vi "judge.vi"(5 "alpha":dbl, 6 "c_y":dbl, 7 "c_x":dbl, 8 "Original Plots":T1(array[cluster]), 9 "dy":dbl, 10 "dx":dbl, 11 "Captured Plots":T1(array[cluster])) -> (0 "result":bool)   [LabVIEW 2012]
panel:
  out "counter":i32
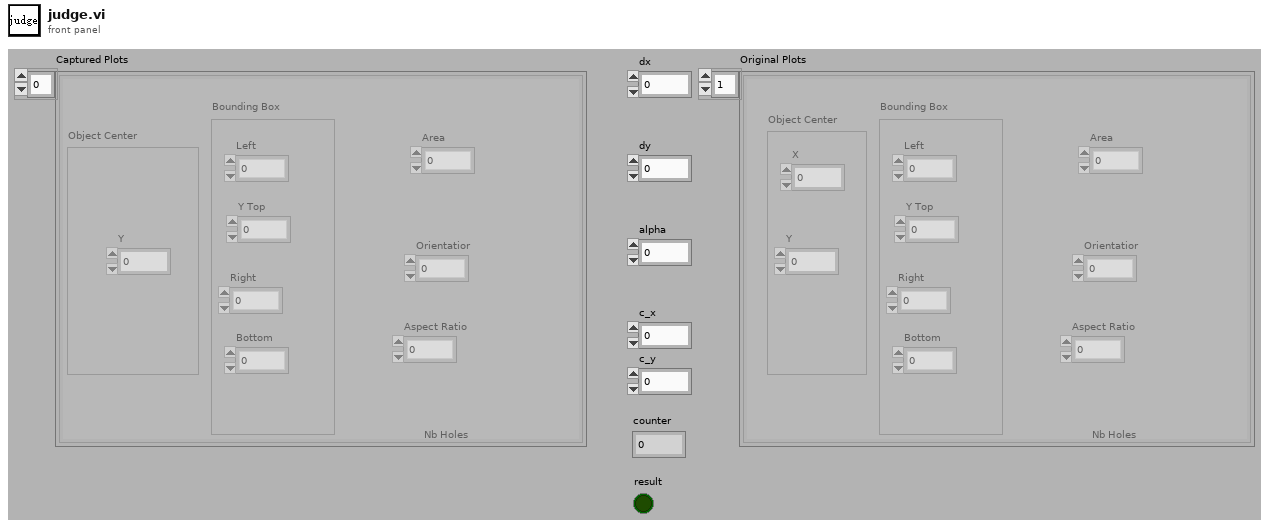
[diagram p1: front panel]
types:
  T1 = cluster{"Object Center":cluster{"X":dbl, "Y":dbl}, "Bounding Box":cluster{"Left":dbl, "Right":dbl, "Bottom":dbl, "Y Top":dbl}, "Area":dbl, "Orientatior":dbl, "Aspect Ratio":dbl, "Nb Holes":dbl}[]
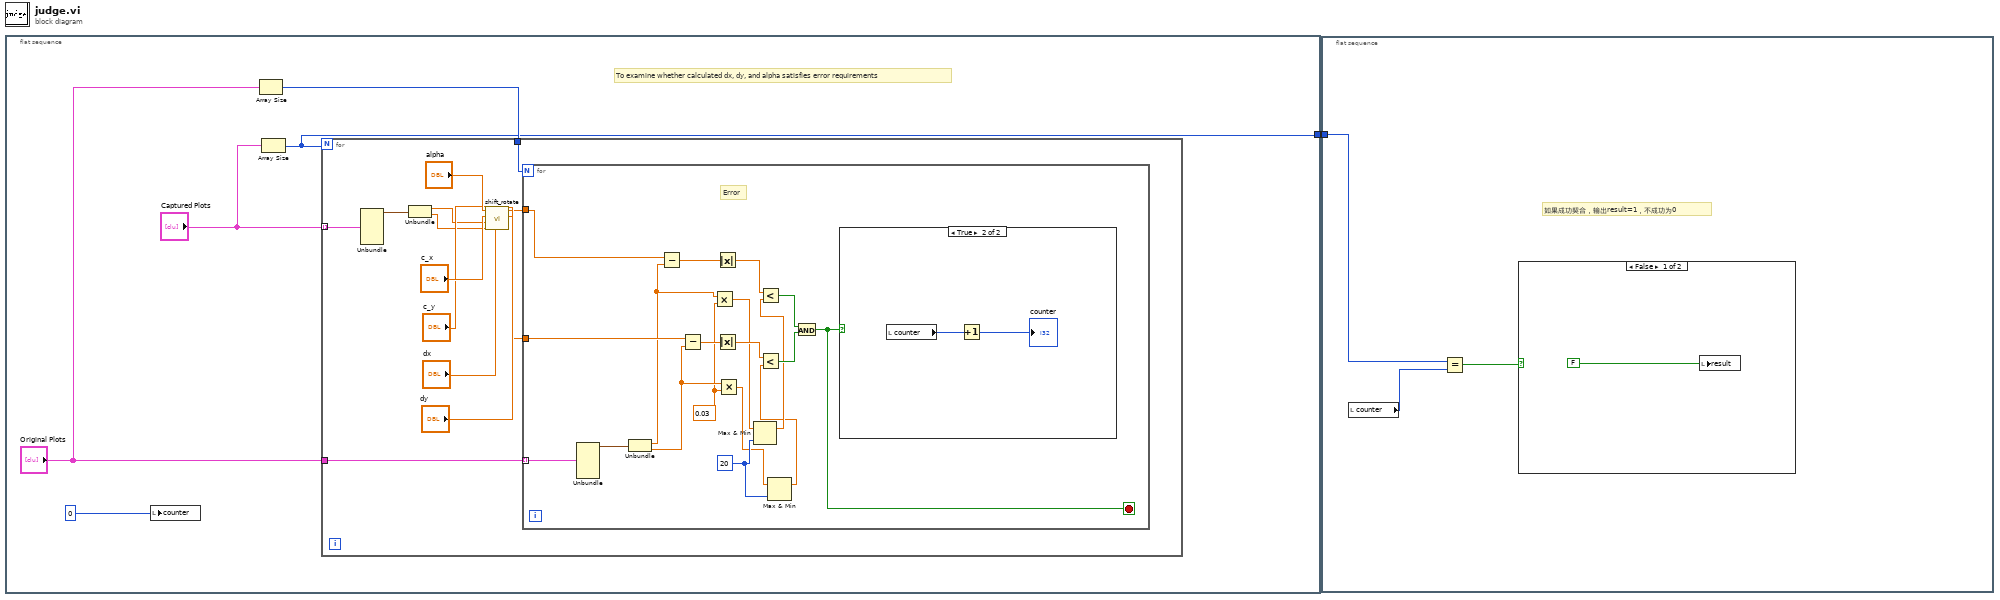
[diagram p0: block diagram]
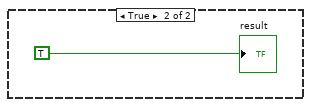
[diagram p2: hidden frame]
diagram:
  n1 = flat-sequence {
    tunnel: [w3] -> w1
    frame #0 {
      # "To examine whether calculated dx, dy, and alpha satisfies error requirements"
      n2 = local write "counter"(0) -> ()
      n3 = Array Size(array="Original Plots") -> (size(s)=w4:i32)
      n4 = Array Size(array="Captured Plots") -> (size(s)=w3:i32)
      n5 = for {
        N: w3 -> [_]
        tunnel: "Captured Plots" -> [w19] mode=indexing
        tunnel: "Original Plots" -> [w10]
        tunnel: w4 -> [w7]
        n6 = Unbundle(w19) -> ("Object Center"=w18:cluster{"X":dbl, "Y":dbl})  [unwired: 5 out]
        n7 = Unbundle(w18) -> ("X"=w14:dbl, "Y"=w13:dbl)
        n8 = call "shift_rotate.vi"("dy"="dy", "dx"="dx", "c_y"="c_y", "y"=w13, "x"=w14, "c_x"="c_x", "alpha"="alpha") -> ("new_y"=w8:dbl, "new_x"=w9:dbl)  [unwired: 3 in]
        n9 = for {
          N: w7 -> [_]
          tunnel: w10 -> [w38] mode=indexing
          tunnel: w9 -> [w28]
          tunnel: w8 -> [w36]
          stop <- w29 stop-if-true
          w24 = 20
          w26 = 0.03 ("y")
          # "Error"
          n10 = Unbundle(w38) -> ("Object Center"=w37:cluster{"X":dbl, "Y":dbl})  [unwired: 5 out]
          n11 = Unbundle(w37) -> ("X"=w25:dbl, "Y"=w27:dbl)
          n12 = Subtract(x=w28, y=w25) -> (x-y=w35:dbl)
          n13 = Subtract(x=w36, y=w27) -> (x-y=w34:dbl)
          n14 = Multiply(x=w25, y=w26) -> (x*y=w23:dbl)
          n15 = Absolute Value(x=w35) -> (abs(x)=w33:dbl)
          n16 = Absolute Value(x=w34) -> (abs(x)=w32:dbl)
          n17 = Multiply(x=w27, y=w26) -> (x*y=w21:dbl)
          n18 = Max & Min(x=w23, y=w24) -> (max(x,y)=w22:dbl)  [unwired: 1 out]
          n19 = Less?(x=w33, y=w22) -> (x < y?=w31:bool)
          n20 = Max & Min(x=w21, y=w24) -> (max(x,y)=w20:dbl)  [unwired: 1 out]
          n21 = Less?(x=w32, y=w20) -> (x < y?=w30:bool)
          n22 = And(x=w31, y=w30) -> (x .and. y?=w29:bool)
          n23 = case shown="True" w29 {
            frame False {
            }
            frame True {
              n24 = local read "counter"() -> (w40:i32)
              n25 = Increment(x=w40) -> (x+1=→"counter":i32)
            }
          }
        }
      }
    }
  }
  n26 = flat-sequence {
    tunnel: w1 -> [w41]
    frame #0 {
      # "如果成功契合，输出result=1，不成功为0"
      n27 = local read "counter"() -> (w42:i32)
      n28 = Equal?(x=w41, y=w42) -> (x = y?=w43:bool)
      n29 = case shown="False" w43 {
        frame False {
          n30 = local write "result"(FALSE) -> ()
        }
        frame True {
          "result" <- TRUE
        }
      }
    }
  }
